vi "Initialize.vi"(7 "Configure RS232 Baud Rate":u32(ring)=9600 items=["9600"=9600, "19200"=19200, "38400"=38400, "57600"=57600, "115200"=115200], 8 "error in (no error)":errorcluster, 9 "Clear Error(True)":bool=TRUE, 10 "ID Query (True)":bool=TRUE, 11 "VISA resource name":refnum<visa-resource-name>) -> (0 "error out":errorcluster, 1 "ID Return Count":i32, 2 "ID Return String":string, 3 "VISA resource name out":refnum<visa-resource-name>)   [LabVIEW 2021, in "GPT-9000.lvlib"]
doc: "Establishes communication with the instrument and optionally performs an instrument identification query and/or an instrument reset. It also places the instrument in a default state needed for other instrument driver operations. Therefore, call this VI before calling other instrument driver VIs for this instrument. Generally, you need to call the Initialize VI only once at the beginning of an application."
uses:
  GPT-9000.lvlib
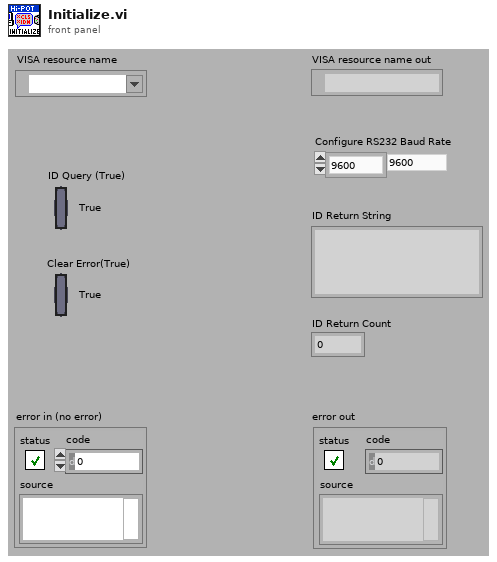
[diagram p1: front panel]
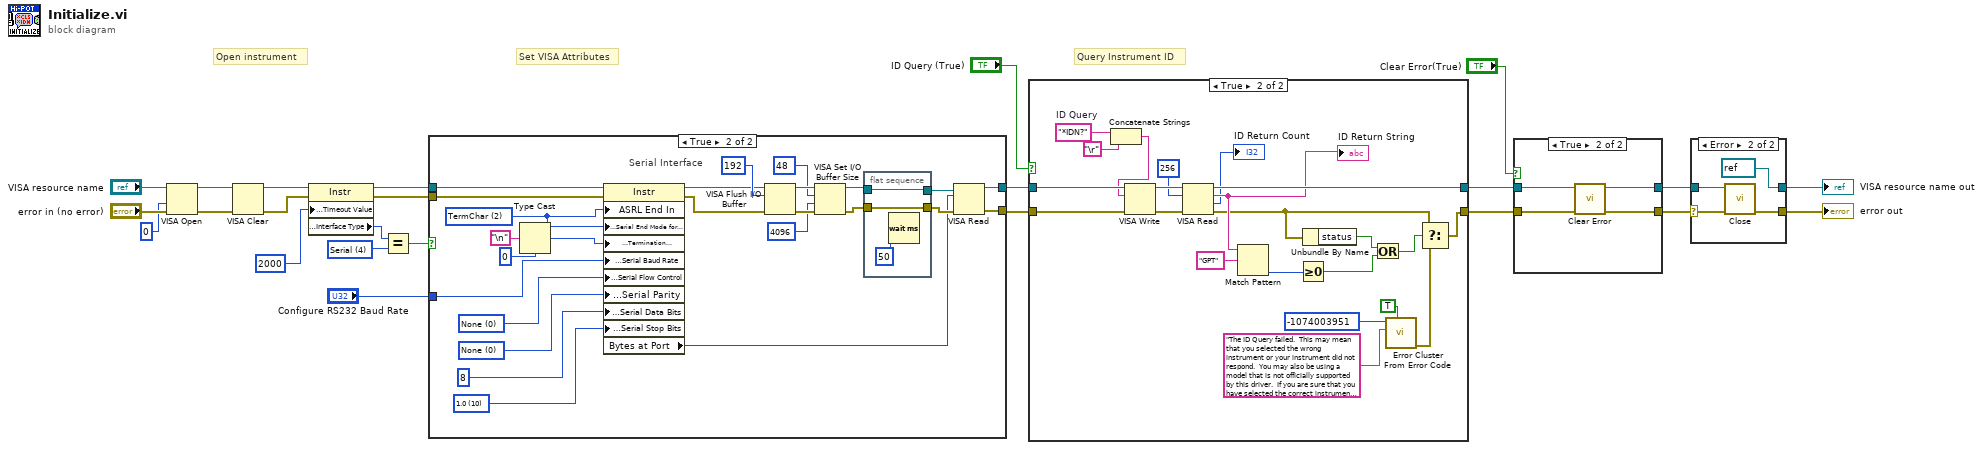
[diagram p0: block diagram]
diagram:
  w12 = u16 4 items=["GPIB"=1, "VXI"=2, "GPIB-VXI"=3, "Serial"=4, "PXI"=5, "TCPIP"=6, "USB"=7] ("Interface Information:Interface Type")
  # "Set VISA Attributes"
  # "Query Instrument ID"
  # "Open instrument"
  n1 = VISA Open(access mode=u32 0, error in (no error)="error in (no error)", VISA resource name="VISA resource name") -> (VISA resource name=w2:refnum<visa-resource-name>, error out=w1:errorcluster)  [unwired: 2 in]
  n2 = VISA Clear(VISA resource name=w2, error in (no error)=w1) -> (VISA resource name out=w10:refnum<visa-resource-name>, error out=w9:errorcluster)
  n3 = property class="Instr"(reference=w10, error in=w9, "General Settings:Timeout Value"=u32 2000) -> (reference out=w15:refnum<visa-resource-name>, error out=w14:errorcluster, "Interface Information:Interface Type"=w18:u16)
  n4 = Equal?(x=w18, y=w12) -> (x = y?=w13:bool)
  n5 = case shown="True" w13 {
    tunnel: [w25 w33] -> w16
    tunnel: [w26 w32] -> w3
    tunnel: w15 -> [w25 w50]
    tunnel: w14 -> [w26 w51]
    tunnel: "Configure RS232 Baud Rate" -> [_ w37]
    frame False {
      # "EDIT: Remove interfaces not\nsupported by your instrument."
      # "GPIB, TCP/IP, and USB Interface"
    }
    frame True {
      w40 = u16 10 items=["1.0"=10, "1.5"=15, "2.0"=20] ("Serial Settings:Stop Bits")
      w38 = u16 0 items=["None", "Odd", "Even", "Mark", "Space"] ("Serial Settings:Parity")
      w39 = u16 0 items=["None", "XON/XOFF", "RTS/CTS", "XON/XOFF & RTS/CTS", "DTR/DSR", "XON/XOFF & DTR/DSR"] ("Serial Settings:Flow Control")
      w36 = u16 2 items=["None", "LastBit", "TermChar"] ("Serial Settings:Serial End Mode for Reads")
      # "Serial Interface"
      n6 = Type Cast(type=u8 0, x="\n") -> (*(type *) &x=w42:u8)
      n7 = property class="Instr"(reference=w50, error in=w51, "ASRL End In"=w36, "Serial Settings:Serial End Mode for Writes"=w36, "Message Based Settings:Termination Character"=w42, "Serial Settings:Serial Baud Rate"=w37, "Serial Settings:Serial Flow Control"=w39, "Serial Settings:Serial Parity"=w38, "Serial Settings:Serial Data Bits"=u16 8 ("Serial Settings:Data Bits"), "Serial Settings:Serial Stop Bits"=w40) -> (reference out=w35:refnum<visa-resource-name>, error out=w34:errorcluster, "Bytes at Port"=w27:u32)
      n8 = VISA Flush I/O Buffer(VISA resource name=w35, mask (16)=u16 192, error in (no error)=w34) -> (VISA resource name out=w49:refnum<visa-resource-name>, error out=w48:errorcluster)
      n9 = VISA Set I/O Buffer Size(VISA resource name=w49, mask (16)=u16 48, size (4096)=u32 4096 ("size (0)"), error in (no error)=w48) -> (VISA resource name out=w31:refnum<visa-resource-name>, error out=w30:errorcluster)
      n10 = flat-sequence {
        tunnel: w31 -> [w54]
        tunnel: w30 -> [w53]
        tunnel: [w54] -> w28
        tunnel: [w53] -> w29
        frame #0 {
          n11 = Wait (ms)(milliseconds to wait=u32 50) -> ()  [unwired: 1 out]
        }
      }
      n12 = VISA Read(VISA resource name=w28, byte count=w27, error in (no error)=w29) -> (VISA resource name out=w33:refnum<visa-resource-name>, error out=w32:errorcluster)  [unwired: 2 out]
    }
  }
  n13 = case shown="True" "ID Query (True)" {
    tunnel: [w55 w78] -> w23
    tunnel: [w56 w75] -> w24
    tunnel: w16 -> [w56 w76]
    tunnel: w3 -> [w55 w77]
    frame False {
    }
    frame True {
      w59 = "*IDN?"  # ID Query
      n14 = Concatenate Strings(w59, "\r" ("string")) -> (w57:string)
      n15 = VISA Write(VISA resource name=w76, write buffer=w57, error in (no error)=w77) -> (VISA resource name out=w74:refnum<visa-resource-name>, error out=w73:errorcluster)  [unwired: 1 out]
      n16 = VISA Read(VISA resource name=w74, byte count=u32 256, error in (no error)=w73) -> (VISA resource name out=w75:refnum<visa-resource-name>, read buffer=w62:string, return count=→"ID Return Count":u32, error out=w60:errorcluster)
      "ID Return String" <- w62
      n17 = Match Pattern(string=w62, regular expression="GPT") -> (offset past match=w66:i32)  [unwired: 1 in, 3 out]
      n18 = Greater Or Equal To 0?(x=w66) -> (x >= 0?=w64:bool)
      n19 = Unbundle By Name(w60) -> ("status"=w65:bool)
      n20 = Or(x=w65, y=w64) -> (x .or. y?=w63:bool)
      n21 = call <vilib>:"Error Cluster From Error Code.vi"("show call chain? (False)"=TRUE, "error message (\"\")"="The ID Query failed.  This may mean that you selected the wrong instrument or your instrument did not respond.  You may also be using a model that is not officially supported by this driver.  If you are sure that you have selected the correct instrument and it is responding, try disabling the ID Query." ("Source (VI Name)"), "error code (0)"=-1074003951 ("Code")) -> ("error out"=w70:errorcluster)  [unwired: 6 in]
      n22 = Select(t=w60, s=w63, f=w70) -> (s? t:f=w78:errorcluster)
    }
  }
  n23 = case shown="True" "Clear Error(True)" {
    tunnel: w23 -> [w79 w84]
    tunnel: [w79 w81] -> w5
    tunnel: w24 -> [w80 w83]
    tunnel: [w80 w82] -> w6
    frame False {
    }
    frame True {
      n24 = call "Clear Error.vi"("error in (no error)"=w84, "VISA resource name"=w83) -> ("error out"=w81:errorcluster, "VISA resource name out"=w82:refnum<visa-resource-name>)  [unwired: 8 in]
    }
  }
  n25 = case shown="Error" w5 {
    selector: w5 -> [w85 w88]
    tunnel: w6 -> [w86 w89]
    tunnel: [w86 refnum<visa-resource-name> refnum ("VISA resource name out")] -> w8
    tunnel: [w85 w90] -> w7
    frame No Error {
    }
    frame Error {
      n26 = call "Close.vi"("error in (no error)"=w88, "VISA resource name"=w89) -> ("error out"=w90:errorcluster)  [unwired: 9 in]
    }
  }
  "VISA resource name out" <- w8
  "error out" <- w7
